vi "Translator.Translate.Event (Single).vi"(8 "error in (no error)":errorcluster, 9 "Arg":variant, 10 "msg":T1) -> (0 "error out":errorcluster, 2 "Translated Msg":string)   [LabVIEW 2019, in "Tools.lvlib"]
uses:
  Tools.lvlib
  Translator.Messages.Event.ctl
  <vilib>/dlg_ctls.llb/Space Constant.vi
  Translator.Global.vi
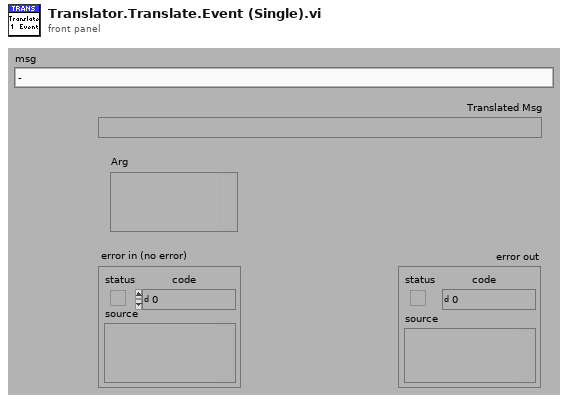
[diagram p1: front panel]
types:
  T1 = typedef "Tools.lvlib/Translator.Messages.Event.ctl" = enum16{"-", "Log out", "Log in", "%s error %d >> %s >> %s", "Starting %s", "Quitting %s", "User %s level %s added", "User %s level %s deleted", "User %s level %s changed to %s"}
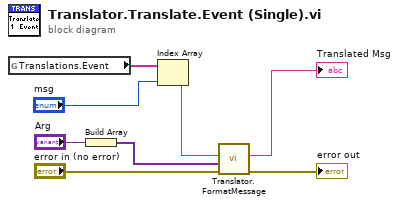
[diagram p0: block diagram]
diagram:
  n1 = global read "Translator.Global.vi" "Translations.Event"() -> (w6:string[])
  n2 = Build Array("Arg") -> (w1:variant[])
  n3 = Index Array(array=w6, index="msg") -> (element=w4:string)
  n4 = call "Translator.FormatMessage.vi"("error in (no error)"="error in (no error)", "Arguments"=w1, "Msg"=w4) -> ("error out"=→"error out":errorcluster, "Translated Msg"=→"Translated Msg":string)  [unwired: 7 in]
